vi "Save Test Vector to file.vi"(8 "error in (no error)":errorcluster, 11 "Test Vector Demo In":refnum<class "Test Vector Demo.lvclass">) -> (0 "error out":errorcluster, 3 "Test Vector Demo Out":refnum<class "Test Vector Demo.lvclass">)   [LabVIEW 2020, in "Test Vector Demo.lvclass"]
doc: "This test method executes the test vector on the VI under test, which all are configured using the methods available. A vector consists of multiple components where each component is a single test. A component is defined by setting control input values and expected results for the component. When the test case is run, controls are reinitialized to default values, the configured inputs are set, the VI is run and the outputs are compared against the expected results."
uses:
  Test Vector Demo.lvclass
  C:/Users/anton/Documents/GitHub/LUnit/source/Framework/Test Vector/LUnit Test Vector.lvclass
  Framework/Test Vector/LUnit Test Vector.lvclass/LUnit Test Vector.ctl
  Framework/Test Vector/LUnit Test Vector.lvclass
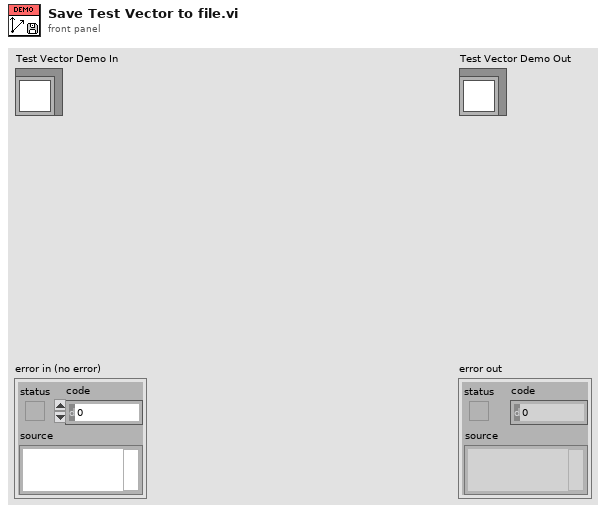
[diagram p1: front panel]
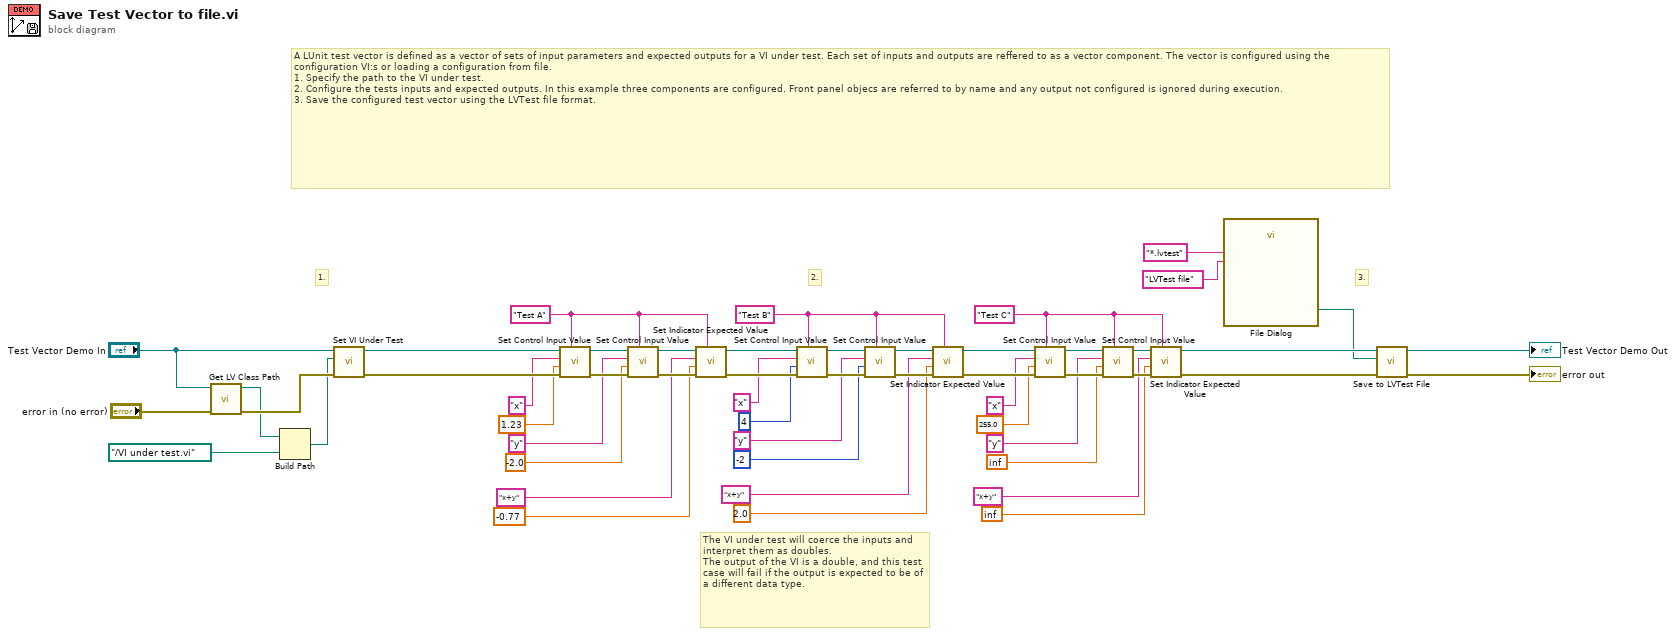
[diagram p0: block diagram]
diagram:
  w8 = "Test C" ("Vector Component")
  w27 = "Test B" ("Vector Component")
  w36 = "Test A" ("Vector Component")
  # "3."
  # "2."
  # "1."
  # "A LUnit test vector is defined as a vector of sets of input parameters and expected outputs for a VI under test. Each set of inputs and outputs are reffered to as a vector component. The vector is configured using the configuration VI:s or loading a configuration from file.\n1. Specify the path to the VI under test.\n2. Configure the tests inputs and expected outputs. In this example three components are configured. Front panel objecs are referred to by name and any output not configured is ignored during execution.\n3. Save the configured test vector using the LVTest file format."
  # "The VI under test will coerce the inputs and interpret them as doubles. \nThe output of the VI is a double, and this test case will fail if the output is expected to be of a different data type."
  n1 = call <vilib>:"Get LV Class Path.vi"("error in (no error)"="error in (no error)", "object"="Test Vector Demo In") -> ("error out"=w16:errorcluster, "class path"=w15:path)  [unwired: 8 in]
  n2 = Build Path(base path=w15, name or relative path=path "../VI under test.vi" ("VI Under Test Path")) -> (appended path=w13:path)
  n3 = call "Set VI Under Test.vi"("error in (no error)"=w16, "VI Under Test Path"=w13, "LUnit Test Vector In"="Test Vector Demo In") -> ("error out"=w51:errorcluster, "LUnit Test Vector Out"=w52:refnum<class "Test Vector Demo.lvclass">)  [unwired: 7 in]
  n4 = call "Set Control Input Value.vi"("Vector Component"=w36, "error in (no error)"=w51, "Data"=1.23, "Control Name"="x", "LUnit Test Vector In"=w52) -> ("error out"=w49:errorcluster, "LUnit Test Vector Out"=w50:refnum<class "Test Vector Demo.lvclass">)  [unwired: 5 in]
  n5 = call "Set Control Input Value.vi"("Vector Component"=w36, "error in (no error)"=w49, "Data"=-2.0, "Control Name"="y", "LUnit Test Vector In"=w50) -> ("error out"=w47:errorcluster, "LUnit Test Vector Out"=w48:refnum<class "Test Vector Demo.lvclass">)  [unwired: 5 in]
  n6 = call "Set Indicator Expected Value.vi"("Vector Component"=w36, "error in (no error)"=w47, "Data"=-0.77, "Control Name"="x+y", "LUnit Test Vector In"=w48) -> ("error out"=w45:errorcluster, "LUnit Test Vector Out"=w46:refnum<class "Test Vector Demo.lvclass">)  [unwired: 5 in]
  n7 = call "Set Control Input Value.vi"("Vector Component"=w27, "error in (no error)"=w45, "Data"=4, "Control Name"="x", "LUnit Test Vector In"=w46) -> ("error out"=w43:errorcluster, "LUnit Test Vector Out"=w44:refnum<class "Test Vector Demo.lvclass">)  [unwired: 5 in]
  n8 = call "Set Control Input Value.vi"("Vector Component"=w27, "error in (no error)"=w43, "Data"=-2, "Control Name"="y", "LUnit Test Vector In"=w44) -> ("error out"=w41:errorcluster, "LUnit Test Vector Out"=w42:refnum<class "Test Vector Demo.lvclass">)  [unwired: 5 in]
  n9 = call "Set Indicator Expected Value.vi"("Vector Component"=w27, "error in (no error)"=w41, "Data"=2.0, "Control Name"="x+y", "LUnit Test Vector In"=w42) -> ("error out"=w39:errorcluster, "LUnit Test Vector Out"=w40:refnum<class "Test Vector Demo.lvclass">)  [unwired: 5 in]
  n10 = call "Set Control Input Value.vi"("Vector Component"=w8, "error in (no error)"=w39, "Data"=255.0, "Control Name"="x", "LUnit Test Vector In"=w40) -> ("error out"=w37:errorcluster, "LUnit Test Vector Out"=w38:refnum<class "Test Vector Demo.lvclass">)  [unwired: 5 in]
  n11 = call "Set Control Input Value.vi"("Vector Component"=w8, "error in (no error)"=w37, "Data"=inf, "Control Name"="y", "LUnit Test Vector In"=w38) -> ("error out"=w11:errorcluster, "LUnit Test Vector Out"=w12:refnum<class "Test Vector Demo.lvclass">)  [unwired: 5 in]
  n12 = call "Set Indicator Expected Value.vi"("Vector Component"=w8, "error in (no error)"=w11, "Data"=inf, "Control Name"="x+y", "LUnit Test Vector In"=w12) -> ("error out"=w5:errorcluster, "LUnit Test Vector Out"=w7:refnum<class "Test Vector Demo.lvclass">)  [unwired: 5 in]
  n13 = call "File Dialog"("pattern (all files)"="*.lvtest", "pattern label"="LVTest file") -> ("selected path"=w2:path)  [unwired: 10 in, 3 out]
  n14 = call "Save to LVTest File.vi"("error in (no error)"=w5, "LVTest File Path"=w2, "LUnit Test Vector In"=w7) -> ("error out"=→"error out":errorcluster, "LUnit Test Vector Out"=→"Test Vector Demo Out":refnum<class "Test Vector Demo.lvclass">)  [unwired: 7 in]
